vi "Form_progr_tareas.vi"() -> ()   [LabVIEW 2017]
uses:
  contador1_global.vi
  contador2_global.vi
  Global_linker_path_3.vi
  <vilib>/addons/database/Connection.llb/DB Tools Open Connec (Path).vi
  global_act_eje_edif.vi
  global_act_eje_aula.vi
  <vilib>/addons/database/_DB Variant To Data/Database Variant To Data.xnode
  <vilib>/addons/database/NI_Database_API.lvlib
  GlobalFag.vi
panel:
  out "serv_ fn":string
  out "serv_":string
  out "serv_s":string
  out "output 1":timestamp
  in  "stop_edificio":bool
  in  "Eliminar":bool
  in  "ID Tarea":u16
  out "Table Control":string[][](table)
  out "Tabla":string
  in  "Tab Control":enum32{"Aula", "Edificio"}(tab)
  in  "+                 -":bool
  in  "edo_actual_aula":bool
  in  "Nota_aula":string
  in  "dias aula":bool[](array[boolean])
  in  "Inicio_aula":timestamp format="%<%x\n%H:%M:%S>T"
  in  "Fin_aula":timestamp format="%<%x\n%H:%M:%S>T"
  in  "Servicios":bool[](array[boolean])
  in  "Edificio":enum8{"A", "B", "C", "D", "E"}(ring)
  in  "Aula":T1(ring)
  in  "Enviar":bool
  out "Loading":bool
  in  "Edificio":enum8{"A", "B", "C", "D", "E"}(ring)
  in  "Servicios_Edif":bool[](array[boolean])
  in  "Fin_edif":timestamp format="%<%x\n%H:%M:%S>T"
  in  "Inicio_edif":timestamp format="%<%x\n%H:%M:%S>T"
  in  "dias_edif":bool[](array[boolean])
  in  "Enviar 3":bool
  in  "rango":bool
  in  "De":u8=1 min=1 max=16
  in  "Hasta":u8=16 min=1 max=16
  in  "edo_actual_aula 2":bool
  in  "+                - 2":bool
  in  "Nota_Edif":string
  # "Programación por Aula"
  # "Notas"
  # "Fecha y hora de inicio - fin"
  # "Fin"
  # "Servicio"
  # "Inicio"
  # "Lunes"
  # "a  Luz"
  # "Martes"
  # "b  Aire"
  # "Miercoles"
  # "+/- Edo. Actual"
  # "Jueves"
  # "c  Proyector"
  # "Viernes"
  # "Sabado"
  # "d  Agua"
  # "Domingo"
  # "e  Acceso"
  # "Programación por Edificio"
  # "Notas"
  # "Fecha y hora de inicio - fin"
  # "Fin"
  # "Servicio"
  # "Inicio"
  # "Lunes"
  # "a  Luz"
  # "Martes"
  # "b  Aire"
  # "Miercoles"
  # "Aplicar a un rango"
  # "Jueves"
  # "c  Proyector"
  # "+/- Edo. Actual"
  # "Viernes"
  # "Sabado"
  # "d  Agua"
  # "Domingo"
  # "e  Acceso"
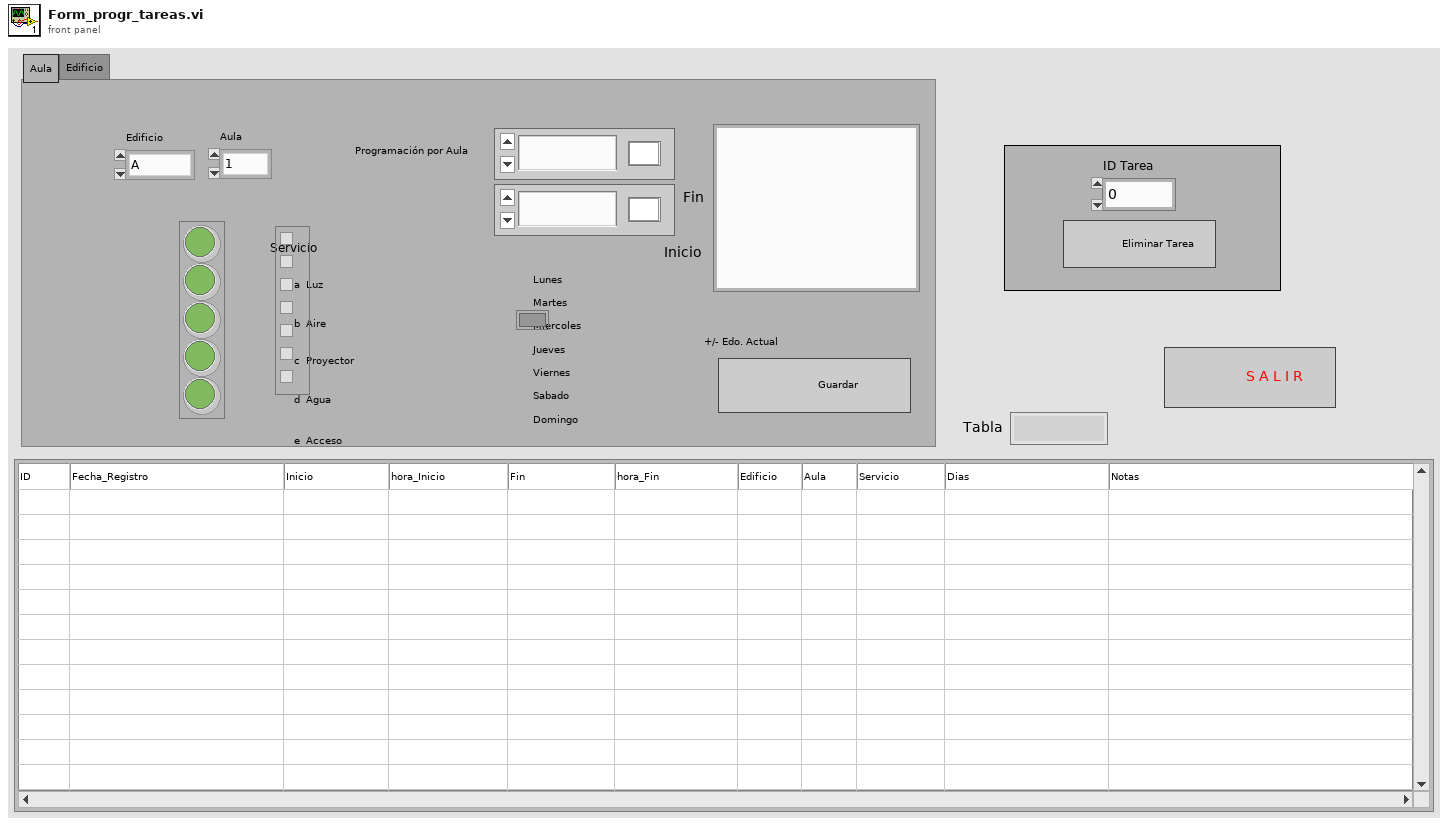
[diagram p1: front panel]
types:
  T1 = enum8{"1", "2", "3", "4", "5", "6", "7", "8", "9", "10", "11", "12", "13", "14", "15", "16"}
  T2 = enum16{"open", "replace", "create", "open or create", "replace or create", "replace or create with confirmation"}
  T3 = typedef "NI_Database_API.lvlib/Conn ObjectReference.ctl" = refnum<k1>
  T4 = cluster{u64, string, "date string":string, "time string":string, "date string":string, "time string":string, string, "string":string, "serv_ fn":string, "dias 2":string, "Nota_Edif":string, string, string, string, "string":string, "string":string, string, string}
  T5 = cluster{u64, string, "date string":string, "time string":string, "date string":string, "time string":string, string, string, "serv_s":string, "dias 2":string, "Nota_aula":string, string, string, string, string, string, string, string}
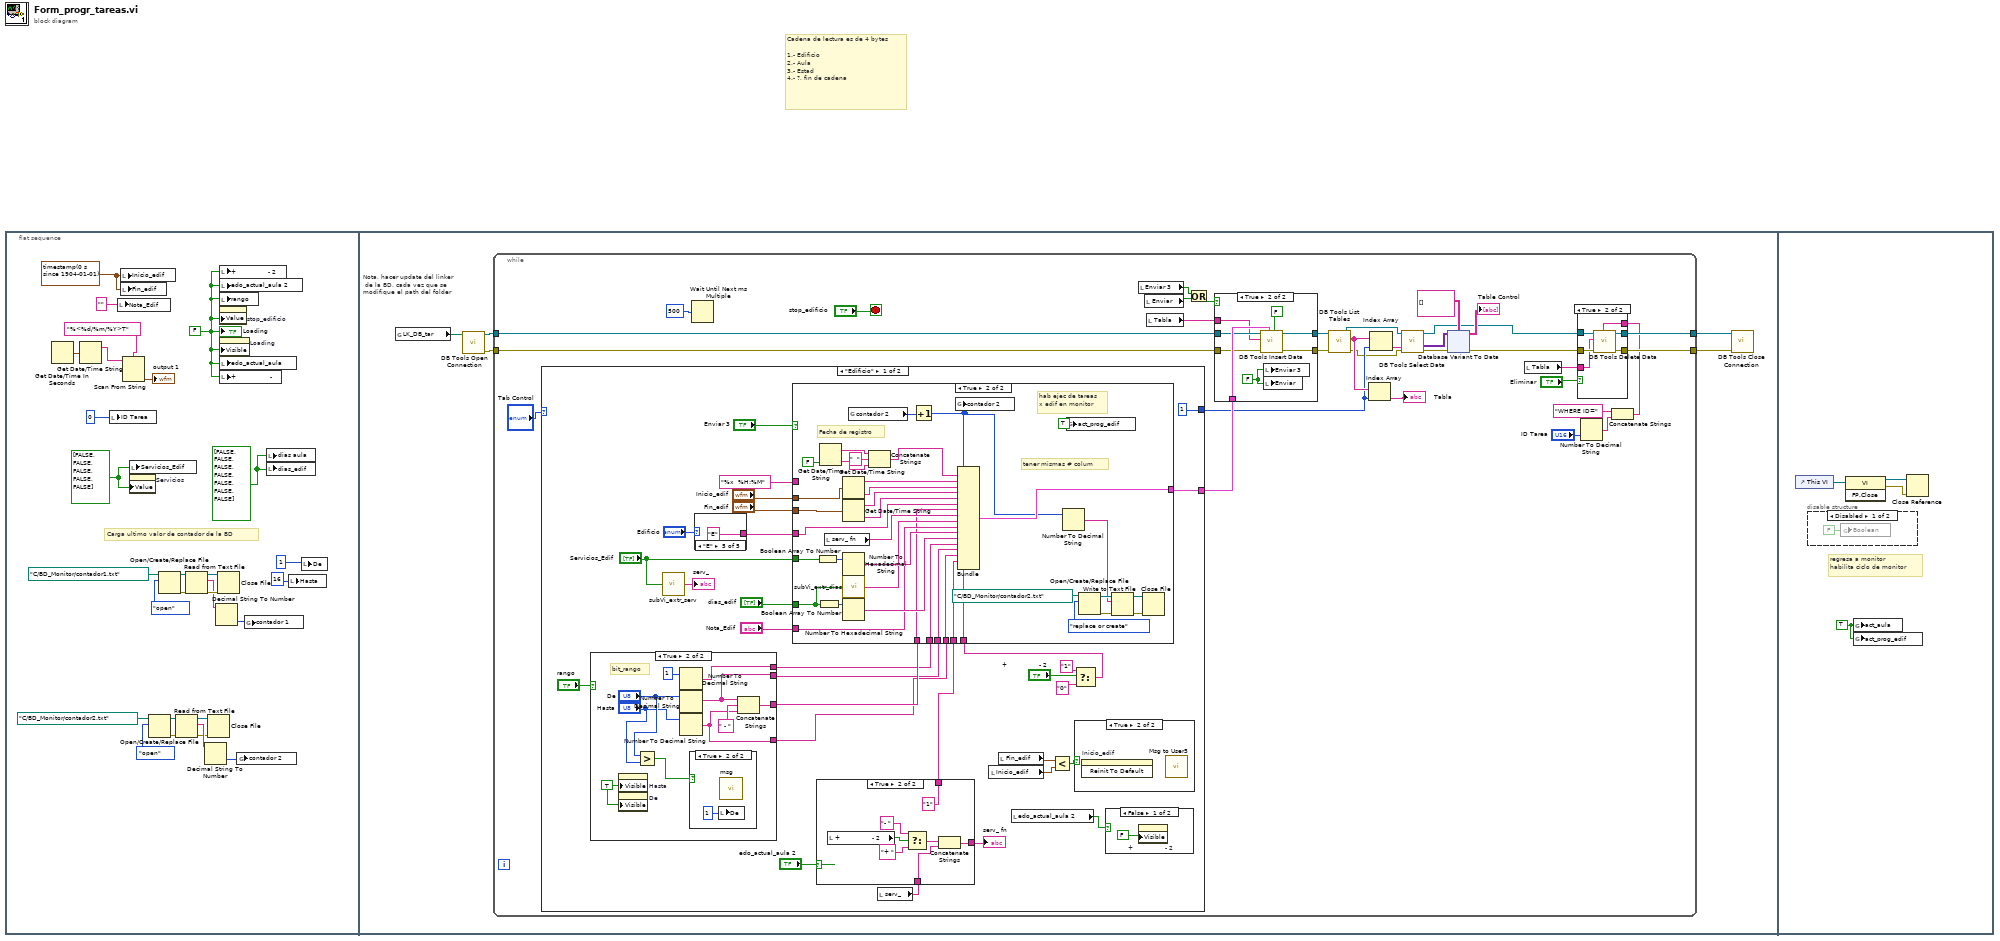
[diagram p0: block diagram]
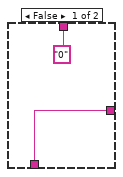
[diagram p4: hidden frame]
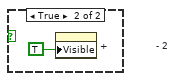
[diagram p5: hidden frame]
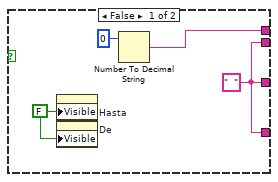
[diagram p6: hidden frame]
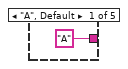
[diagram p9: hidden frame]
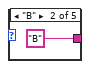
[diagram p10: hidden frame]
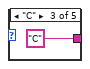
[diagram p11: hidden frame]
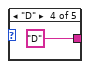
[diagram p12: hidden frame]
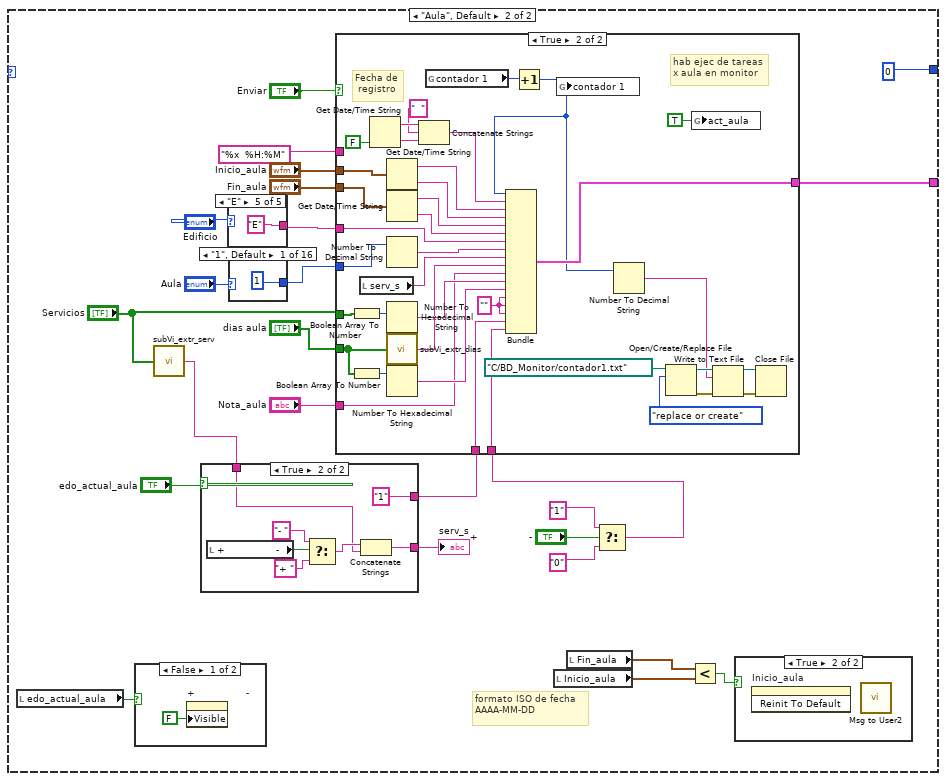
[diagram p14: hidden frame]
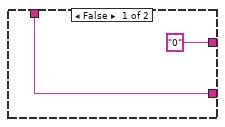
[diagram p15: hidden frame]
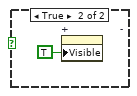
[diagram p16: hidden frame]
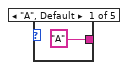
[diagram p18: hidden frame]
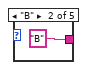
[diagram p19: hidden frame]
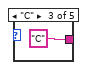
[diagram p20: hidden frame]
diagram:
  # "Cadena de lectura es de 4 bytes\n\n1.- Edificio\n2.- Aula\n3.- Estad\n4.- ?, fin de cadena"
  n1 = flat-sequence {
    frame #0 {
      w3 = timestamp(0 s since 1904-01-01) ("Inicio_edif")
      w28 = bool[] [FALSE, FALSE, FALSE, FALSE, FALSE, FALSE, FALSE] ("Servicios 2")
      w8 = FALSE ("Loading")
      w27 = bool[] [FALSE, FALSE, FALSE, FALSE, FALSE] ("Servicios")
      # "Carga ultimo valor de contador de la BD"
      n2 = Get Date/Time In Seconds() -> (seconds since 1Jan1904=w7:timestamp)
      n3 = Get Date/Time String(seconds (now)=w7) -> (date string=w6:string)  [unwired: 2 in, 1 out]
      n4 = local write "ID Tarea"(u16 0) -> ()
      n5 = local write "Nota_Edif"("") -> ()
      n6 = local write "Inicio_edif"(w3) -> ()
      n7 = local write "Fin_edif"(w3) -> ()
      n8 = Scan From String(format string="%<%d/%m/%Y>T", input string=w6) -> (output 1=→"output 1":timestamp)  [unwired: 3 in, 3 out]
      n9 = local write "Servicios_Edif"(w27) -> ()
      n10 = property on="Servicios" class="Arr (strict)"("Value"=w27) -> ()  [unwired: 2 in, 2 out]
      n11 = Open/Create/Replace File(file path (use dialog)=path "C:/BD_Monitor/contador2.txt" ("path"), operation (0:open)=T2."open") -> (refnum out=w17:refnum<file>, error out=w18:errorcluster)  [unwired: 4 in, 1 out]
      n12 = Open/Create/Replace File(file path (use dialog)=path "C:/BD_Monitor/contador1.txt" ("path"), operation (0:open)=T2."open") -> (refnum out=w23:refnum<file>, error out=w22:errorcluster)  [unwired: 4 in, 1 out]
      n13 = Read from Text File(file (use dialog)=w17, error in=w18) -> (refnum out=w16:refnum<file>, text=w19:string, error out=w15:errorcluster)  [unwired: 2 in, 1 out]
      n14 = Read from Text File(file (use dialog)=w23, error in=w22) -> (refnum out=w24:refnum<file>, text=w21:string, error out=w25:errorcluster)  [unwired: 2 in, 1 out]
      n15 = Decimal String To Number(string=w19) -> (number=w13:i32)  [unwired: 2 in, 1 out]
      n16 = Close File(refnum=w16, error in=w15) -> ()  [unwired: 2 out]
      n17 = Decimal String To Number(string=w21) -> (number=w20:i32)  [unwired: 2 in, 1 out]
      n18 = Close File(refnum=w24, error in=w25) -> ()  [unwired: 2 out]
      n19 = local write "+                - 2"(w8) -> ()
      n20 = local write "edo_actual_aula 2"(w8) -> ()
      n21 = local write "rango"(w8) -> ()
      n22 = property on="stop_edificio" class="Bool (strict)"("Value"=w8) -> ()  [unwired: 2 in, 2 out]
      n23 = property on="Loading" class="Bool (strict)"("Visible"=w8) -> ()  [unwired: 2 in, 2 out]
      n24 = local write "edo_actual_aula"(w8) -> ()
      n25 = local write "+                 -"(w8) -> ()
      n26 = global write "contador2_global.vi" "contador 2"(w13) -> ()
      n27 = global write "contador1_global.vi" "contador 1"(w20) -> ()
      n28 = local write "dias aula"(w28) -> ()
      n29 = local write "dias_edif"(w28) -> ()
      n30 = local write "Hasta"(u8 16) -> ()
      n31 = local write "De"(u8 1) -> ()
      "Loading" <- w8
    }
    frame #1 {
      # "Nota, hacer update del linker\n de la BD, cada vez que se \nmodifique el path del folder"
      n32 = global read "Global_linker_path_3.vi" "LK_DB_tar"() -> (w29:path)
      n33 = call-poly <vilib>:"DB Tools Open Connection.vi"("connection information"=w29) -> ("error out"=w33:errorcluster, "connection reference"=w32:T3)  [unwired: 7 in]
      n34 = while {
        tunnel: w33 -> [w62]
        tunnel: w32 -> [w61]
        tunnel: [w42] -> w31
        tunnel: [w41] -> w30
        stop <- "stop_edificio" stop-if-true
        n35 = case shown="\"Edificio\"" "Tab Control" {
          tunnel: [w144 w230] -> w63
          tunnel: [1 0] -> w48
          frame "Edificio" {
            n36 = case shown="True" "rango" {
              tunnel: [w168 w180] -> w141
              tunnel: [w169 w176] -> w140
              tunnel: [w168 w172] -> w139
              tunnel: [w168 w178] -> w138
              frame False {
                w171 = FALSE ("Visible")
                w168 = "  " ("string")
                n37 = property on="Hasta" class="DigNum (strict)"("Visible"=w171) -> ()  [unwired: 2 in, 2 out]
                n38 = property on="De" class="DigNum (strict)"("Visible"=w171) -> ()  [unwired: 2 in, 2 out]
                n39 = Number To Decimal String(number=u8 0) -> (decimal integer string=w169:string)  [unwired: 1 in]
              }
              frame True {
                w179 = TRUE ("Visible")
                # "bit_rango"
                n40 = property on="Hasta" class="DigNum (strict)"("Visible"=w179) -> ()  [unwired: 2 in, 2 out]
                n41 = property on="De" class="DigNum (strict)"("Visible"=w179) -> ()  [unwired: 2 in, 2 out]
                n42 = Greater?(x="De", y="Hasta") -> (0:w173:bool)
                n43 = Number To Decimal String(number=u8 1) -> (decimal integer string=w176:string)  [unwired: 1 in]
                n44 = Number To Decimal String(number="De") -> (decimal integer string=w172:string)  [unwired: 1 in]
                n45 = Number To Decimal String(number="Hasta") -> (decimal integer string=w178:string)  [unwired: 1 in]
                n46 = case shown="True" w173 {
                  frame False {
                  }
                  frame True {
                    n47 = local write "De"(u8 1 ("De")) -> ()
                    n48 = call "msg"() -> ()  [unwired: 10 in, 2 out]
                  }
                }
                n49 = Concatenate Strings(w172, " - ", w178) -> (w180:string)
              }
            }
            n50 = call "subVi_extr_serv.vi"("Servicios_Edif"="Servicios_Edif") -> ("serv"=→"serv_":string)
            n51 = case shown="\"E\"" "Edificio" {
              tunnel: ["A" "B" "C" "D" "E"] -> w151
              frame "A", Default {
              }
              frame "B" {
              }
              frame "C" {
              }
              frame "D" {
              }
              frame "E" {
              }
            }
            n52 = local read "serv_"() -> (w130:string)
            n53 = case shown="True" "edo_actual_aula 2" {
              tunnel: [w158 w161] -> w128
              tunnel: w130 -> [w158 w160]
              tunnel: ["0" "1"] -> w129
              frame False {
              }
              frame True {
                n54 = local read "+                - 2"() -> (w165:bool)
                n55 = Select(t="- ", s=w165, f="+ ") -> (s? t:f=w162:string)
                n56 = Concatenate Strings(w162, w160) -> (w161:string)
              }
            }
            "serv_ fn" <- w128
            n57 = local read "Inicio_edif"() -> (w148:timestamp)
            n58 = local read "Fin_edif"() -> (w149:timestamp)
            n59 = local read "edo_actual_aula 2"() -> (w134:bool)
            n60 = Less?(x=w149, y=w148) -> (x < y?=w150:bool)
            n61 = Select(t="1", s="+                - 2", f="0") -> (s? t:f=w133:string)
            n62 = case shown="True" "Enviar 3" {
              tunnel: "Servicios_Edif" -> [_ w208]
              tunnel: "Inicio_edif" -> [_ w206]
              tunnel: "Fin_edif" -> [_ w203]
              tunnel: "%x  %H:%M" ("time format string (%c)") -> [_ _]
              tunnel: "dias_edif" -> [_ w207]
              tunnel: w151 -> [_ w200]
              tunnel: [_ w220] -> w144
              tunnel: "Nota_Edif" -> [_ w199]
              tunnel: w141 -> [_ w189]
              tunnel: w140 -> [_ w197]
              tunnel: w139 -> [_ w196]
              tunnel: w138 -> [_ w195]
              tunnel: w129 -> [_ w193]
              tunnel: w133 -> [_ w192]
              frame False {
              }
              frame True {
                # "hab ejec de tareas\nx edif en monitor"
                # "tener mismas # colum"
                # "Fecha de registro"
                n63 = Boolean Array To Number(Boolean array=w208) -> (number=w219:u8)
                n64 = Boolean Array To Number(Boolean array=w207) -> (number=w218:u8)
                n65 = Get Date/Time String(want seconds? (F)=FALSE) -> (date string=w225:string, time string=w222:string)  [unwired: 2 in]
                n66 = local read "serv_ fn"() -> (w190:string)
                n67 = Get Date/Time String(seconds (now)=w206) -> (date string=w205:string, time string=w204:string)  [unwired: 2 in]
                n68 = Get Date/Time String(seconds (now)=w203) -> (date string=w202:string, time string=w201:string)  [unwired: 2 in]
                n69 = Number To Hexadecimal String(2:w219) -> (0:w210:string)  [unwired: 1 in]
                n70 = call "subVi_extr_dias.vi"("dias_edif 2"=w207) -> ("dias 2"=w194:string)
                n71 = Number To Hexadecimal String(2:w218) -> (0:w209:string)  [unwired: 1 in]
                n72 = global read "contador2_global.vi" "contador 2"() -> (w217:u64)
                n73 = Concatenate Strings(w225, "  " ("string"), w222) -> (w221:string)
                n74 = Increment(x=w217) -> (x+1=w198:u64)
                n75 = global write "contador2_global.vi" "contador 2"(w198) -> ()
                n76 = Bundle(w198, w221, "date string"=w205, "time string"=w204, "date string"=w202, "time string"=w201, w200, "string"=w189, "serv_ fn"=w190, "dias 2"=w194, "Nota_Edif"=w199, w210, w209, w197, "string"=w196, "string"=w195, w193, w192) -> (w220:T4)  [unwired: 1 in]
                n77 = Number To Decimal String(number=w198) -> (decimal integer string=w211:string)  [unwired: 1 in]
                n78 = global write "global_act_eje_edif.vi" "act_prog_edif"(TRUE ("Boolean")) -> ()
                n79 = Open/Create/Replace File(file path (use dialog)=path "C:/BD_Monitor/contador2.txt" ("path"), operation (0:open)=T2."replace or create") -> (refnum out=w214:refnum<file>, error out=w213:errorcluster)  [unwired: 4 in, 1 out]
                n80 = Write to Text File(file (use dialog)=w214, text=w211, error in=w213) -> (refnum out=w216:refnum<file>, error out=w215:errorcluster)  [unwired: 1 in, 1 out]
                n81 = Close File(refnum=w216, error in=w215) -> ()  [unwired: 2 out]
              }
            }
            n82 = case shown="True" w150 {
              frame False {
              }
              frame True {
                n83 = invoke on="Inicio_edif" class="AbsTime (strict)" method="Reinit To Default"() -> ()  [unwired: 3 in, 3 out]
                n84 = call "Msg to User3"() -> ()  [unwired: 10 in, 2 out]
              }
            }
            n85 = case shown="False" w134 {
              frame False {
                n86 = property on="+                - 2" class="Bool (strict)"("Visible"=FALSE ("+                - 2")) -> ()  [unwired: 2 in, 2 out]
              }
              frame True {
                n87 = property on="+                - 2" class="Bool (strict)"("Visible"=TRUE ("+                - 2")) -> ()  [unwired: 2 in, 2 out]
              }
            }
          }
          frame "Aula", Default {
            # "formato ISO de fecha\nAAAA-MM-DD"
            n88 = local read "edo_actual_aula"() -> (w235:bool)
            n89 = case shown="False" w235 {
              frame False {
                n90 = property on="+                 -" class="Bool (strict)"("Visible"=FALSE) -> ()  [unwired: 2 in, 2 out]
              }
              frame True {
                n91 = property on="+                 -" class="Bool (strict)"("Visible"=TRUE) -> ()  [unwired: 2 in, 2 out]
              }
            }
            n92 = call "subVi_extr_serv.vi"("Servicios_Edif"="Servicios") -> ("serv"=w232:string)
            n93 = case shown="True" "edo_actual_aula" {
              tunnel: ["0" "1"] -> w234
              tunnel: w232 -> [w251 w254]
              tunnel: [w251 w253] -> w231
              frame False {
              }
              frame True {
                n94 = local read "+                 -"() -> (w258:bool)
                n95 = Select(t="- ", s=w258, f="+ ") -> (s? t:f=w255:string)
                n96 = Concatenate Strings(w255, w254) -> (w253:string)
              }
            }
            "serv_s" <- w231
            n97 = case shown="\"E\"" "Edificio" {
              tunnel: ["A" "B" "C" "D" "E"] -> w247
              frame "A", Default {
              }
              frame "B" {
              }
              frame "C" {
              }
              frame "D" {
              }
              frame "E" {
              }
            }
            n98 = case shown="\"1\", Default" "Aula" {
              tunnel: [u8 1 u8 2 u8 3 u8 4 u8 5 u8 6 u8 7 u8 8 u8 9 u8 10 u8 11 u8 12 u8 13 u8 14 u8 15 u8 16] -> w243
              frame "1", Default {
              }
              frame "2" {
              }
              frame "3" {
              }
              frame "4" {
              }
              frame "5" {
              }
              frame "6" {
              }
              frame "7" {
              }
              frame "8" {
              }
              frame "9" {
              }
              frame "10" {
              }
              frame "11" {
              }
              frame "12" {
              }
              frame "13" {
              }
              frame "14" {
              }
              frame "15" {
              }
              frame "16" {
              }
            }
            n99 = local read "Inicio_aula"() -> (w244:timestamp)
            n100 = local read "Fin_aula"() -> (w245:timestamp)
            n101 = Select(t="1", s="+                 -", f="0") -> (s? t:f=w227:string)
            n102 = case shown="True" "Enviar" {
              tunnel: w247 -> [_ w319]
              tunnel: w243 -> [_ w312]
              tunnel: "Servicios" -> [_ w299]
              tunnel: "dias aula" -> [_ w298]
              tunnel: "%x  %H:%M" ("time format string (%c)") -> [_ _]
              tunnel: "Inicio_aula" -> [_ w296]
              tunnel: "Fin_aula" -> [_ w295]
              tunnel: [_ w313] -> w230
              tunnel: "Nota_aula" -> [_ w290]
              tunnel: w234 -> [_ w287]
              tunnel: w227 -> [_ w286]
              frame False {
              }
              frame True {
                w288 = ""
                # "hab ejec de tareas\nx aula en monitor"
                # "Fecha de\n registro"
                n103 = Boolean Array To Number(Boolean array=w299) -> (number=w310:u8)
                n104 = Boolean Array To Number(Boolean array=w298) -> (number=w309:u8)
                n105 = local read "serv_s"() -> (w284:string)
                n106 = Get Date/Time String(want seconds? (F)=FALSE) -> (date string=w318:string, time string=w314:string)  [unwired: 2 in]
                n107 = Get Date/Time String(seconds (now)=w296) -> (date string=w294:string, time string=w293:string)  [unwired: 2 in]
                n108 = Get Date/Time String(seconds (now)=w295) -> (date string=w292:string, time string=w291:string)  [unwired: 2 in]
                n109 = Number To Decimal String(number=w312) -> (decimal integer string=w311:string)  [unwired: 1 in]
                n110 = Number To Hexadecimal String(2:w310) -> (0:w301:string)  [unwired: 1 in]
                n111 = call "subVi_extr_dias.vi"("dias_edif 2"=w298) -> ("dias 2"=w297:string)
                n112 = Number To Hexadecimal String(2:w309) -> (0:w300:string)  [unwired: 1 in]
                n113 = Concatenate Strings(w318, "  " ("string"), w314) -> (w315:string)
                n114 = global read "contador1_global.vi" "contador 1"() -> (w308:u64)
                n115 = Increment(x=w308) -> (x+1=w289:u64)
                n116 = Bundle(w289, w315, "date string"=w294, "time string"=w293, "date string"=w292, "time string"=w291, w319, w311, "serv_s"=w284, "dias 2"=w297, "Nota_aula"=w290, w301, w300, w288, w288, w288, w287, w286) -> (w313:T5)  [unwired: 1 in]
                n117 = global write "contador1_global.vi" "contador 1"(w289) -> ()
                n118 = Number To Decimal String(number=w289) -> (decimal integer string=w302:string)  [unwired: 1 in]
                n119 = Open/Create/Replace File(file path (use dialog)=path "C:/BD_Monitor/contador1.txt" ("path"), operation (0:open)=T2."replace or create") -> (refnum out=w305:refnum<file>, error out=w304:errorcluster)  [unwired: 4 in, 1 out]
                n120 = global write "global_act_eje_aula.vi" "act_aula"(TRUE ("act_aula")) -> ()
                n121 = Write to Text File(file (use dialog)=w305, text=w302, error in=w304) -> (refnum out=w307:refnum<file>, error out=w306:errorcluster)  [unwired: 1 in, 1 out]
                n122 = Close File(refnum=w307, error in=w306) -> ()  [unwired: 2 out]
              }
            }
            n123 = Less?(x=w245, y=w244) -> (x < y?=w246:bool)
            n124 = case shown="True" w246 {
              frame False {
              }
              frame True {
                n125 = invoke on="Inicio_aula" class="AbsTime (strict)" method="Reinit To Default"() -> ()  [unwired: 3 in, 3 out]
                n126 = call "Msg to User2"() -> ()  [unwired: 10 in, 2 out]
              }
            }
          }
        }
        n127 = Wait Until Next ms Multiple(millisecond multiple=u32 500) -> ()  [unwired: 1 out]
        n128 = local read "Enviar 3"() -> (w58:bool)
        n129 = local read "Enviar"() -> (w57:bool)
        n130 = local read "Tabla"() -> (w60:string)
        n131 = Or(x=w58, y=w57) -> (x .or. y?=w59:bool)
        n132 = case shown="True" w59 {
          tunnel: w63 -> [_ w127]
          tunnel: w62 -> [w118 w126]
          tunnel: w61 -> [w119 w125]
          tunnel: w60 -> [_ w123]
          tunnel: [w118 w121] -> w56
          tunnel: [w119 w120] -> w55
          frame False {
          }
          frame True {
            w122 = FALSE ("create table? (F)")
            n133 = call <vilib>:"DB Tools Insert Data.vi"("create table? (F)"=FALSE, "data"=w127, "error in (no error)"=w126, "table"=w123, "connection reference"=w125) -> ("error out"=w121:errorcluster, "connection reference out"=w120:T3)  [unwired: 5 in]
            n134 = local write "Enviar 3"(w122) -> ()
            n135 = local write "Enviar"(w122) -> ()
          }
        }
        n136 = call <vilib>:"DB Tools List Tables.vi"("error in (no error)"=w56, "connection reference"=w55) -> ("error out"=w46:errorcluster, "tables"=w53:string[], "connection reference out"=w45:T3)  [unwired: 3 in]
        n137 = Index Array(array=w53, index=w48) -> (element=→"Tabla":string)
        n138 = Index Array(array=w53, index=w48) -> (element=w52:string)
        n139 = call <vilib>:"DB Tools Select Data.vi"("error in (no error)"=w46, "table"=w52, "connection reference"=w45) -> ("error out"=w50:errorcluster, "data"=w51:variant[][], "connection reference out"=w43:T3)  [unwired: 3 in]
        n140 = xnode "Database Variant To Data"("database variant"=w51, "error in (no error)"=w50, "type"=string[][] []) -> ("data"=→"Table Control":string[][], "error out"=w44:errorcluster)
        n141 = local read "Tabla"() -> (w39:string)
        n142 = Number To Decimal String(number="ID Tarea") -> (decimal integer string=w36:string)  [unwired: 1 in]
        n143 = Concatenate Strings("WHERE ID=", w36) -> (w35:string)
        n144 = case shown="True" "Eliminar" {
          tunnel: w44 -> [w66 w73]
          tunnel: w43 -> [w67 w72]
          tunnel: [w66 w71] -> w42
          tunnel: [w67 w70] -> w41
          tunnel: w39 -> [_ w69]
          tunnel: w35 -> [_ w68]
          frame False {
          }
          frame True {
            n145 = call <vilib>:"DB Tools Delete Data.vi"("condition"=w68, "error in (no error)"=w73, "table"=w69, "connection reference"=w72) -> ("error out"=w71:errorcluster, "connection reference out"=w70:T3)  [unwired: 6 in]
          }
        }
      }
      n146 = call <vilib>:"DB Tools Close Connection.vi"("error in (no error)"=w31, "connection reference"=w30) -> ()  [unwired: 5 in, 1 out]
    }
    frame #2 {
      w320 = TRUE ("act_aula")
      # "regresa a monitor\nhabilita ciclo de monitor"
      n147 = control-ref of="This VI"() -> (w321:refnum<vi>)
      n148 = disable-structure shown="Disabled" {
        frame Disabled {
          n149 = global write "GlobalFag.vi" "Boolean"(FALSE ("Boolean")) -> ()
        }
        frame Enabled {
        }
      }
      n150 = invoke class="VI" method="FP.Close"(reference=w321) -> (reference out=w323:refnum<vi>, error out=w322:errorcluster)  [unwired: 2 in, 1 out]
      n151 = global write "global_act_eje_aula.vi" "act_aula"(w320) -> ()
      n152 = global write "global_act_eje_edif.vi" "act_prog_edif"(w320) -> ()
      n153 = Close Reference(reference=w323, error in (no error)=w322) -> ()  [unwired: 1 out]
    }
  }
